vi "Executable Version.vi"() -> ()   [LabVIEW 2014]
panel:
  out "Version of Executable":string
  # "Cut and Paste code from the block diagram  \njust before you build the exectable. Remember \nthis code will give you an error if you try to run\n your program without building it into an executable."
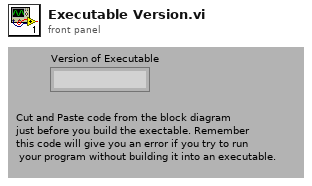
[diagram p1: front panel]
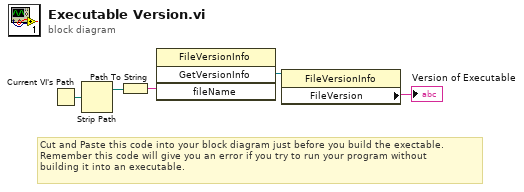
[diagram p0: block diagram]
diagram:
  # "Cut and Paste this code into your block diagram just before you build the exectable.\nRemember this code will give you an error if you try to run your program without\nbuilding it into an executable."
  n1 = Current VI's Path() -> (path=w2:path)
  n2 = Strip Path(path=w2) -> (stripped path=w1:path)  [unwired: 1 out]
  n3 = Path To String(path=w1) -> (string=w5:string)
  n4 = invoke class="FileVersionInfo" method="GetVersionInfo"("fileName"=w5) -> ("GetVersionInfo"=w4:refnum<k24>)  [unwired: 3 in, 3 out]
  n5 = property class="FileVersionInfo"(reference=w4) -> ("FileVersion"=→"Version of Executable":string)  [unwired: 1 in, 2 out]
